vi "Selcol.vi"(10 "Array in":dbl[][](array[numeric]), 11 "Selected":bool[](array[boolean])) -> (3 "Array out":dbl[][](array[numeric]))   [LabVIEW 2014]
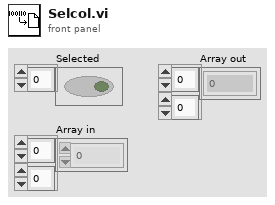
[diagram p1: front panel]
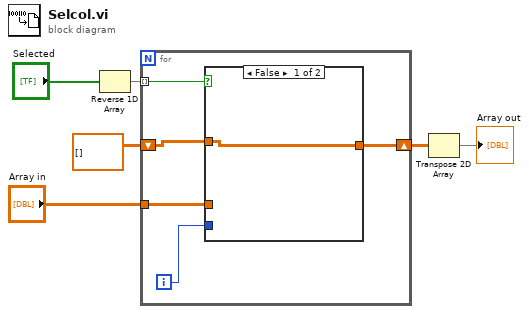
[diagram p0: block diagram]
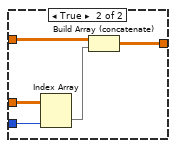
[diagram p2: hidden frame]
diagram:
  n1 = Reverse 1D Array(array="Selected") -> (reversed array=w6:bool[])
  n2 = for {
    tunnel: w6 -> [w11] mode=indexing
    tunnel: "Array in" -> [w10]
    shift-right: [w8] -> w4
    shift-left: dbl[][] [] -> [w7]
    i -> [w9]
    n3 = case shown="False" w11 {
      tunnel: w10 -> [_ w17]
      tunnel: w9 -> [_ w16]
      tunnel: [w12 w14] -> w8
      tunnel: w7 -> [w12 w13]
      frame False {
      }
      frame True {
        n4 = Index Array(array=w17, index (col)=w16) -> (element=w15:dbl[])  [unwired: 1 in]
        n5 = Build Array (concatenate)(w13, w15) -> (w14:dbl[][])
      }
    }
  }
  n6 = Transpose 2D Array(2D array=w4) -> (transposed array=→"Array out":dbl[][])
